vi "B_WriteClassAttribute.vi"(8 "error in (no error)":errorcluster, 11 "reference in":refnum<class "BaseTemplate_4x4x4.lvclass">) -> (0 "error out":errorcluster, 3 "reference out":refnum<class "BaseTemplate_4x4x4.lvclass">)   [LabVIEW 2012]
uses:
  <resource>/Framework/Providers/Open_GDS/ClassProviders/Provider_EndevoGOOP300/Templates/BaseTemplate_4x4x4/BaseTemplate_4x4x4.lvclass
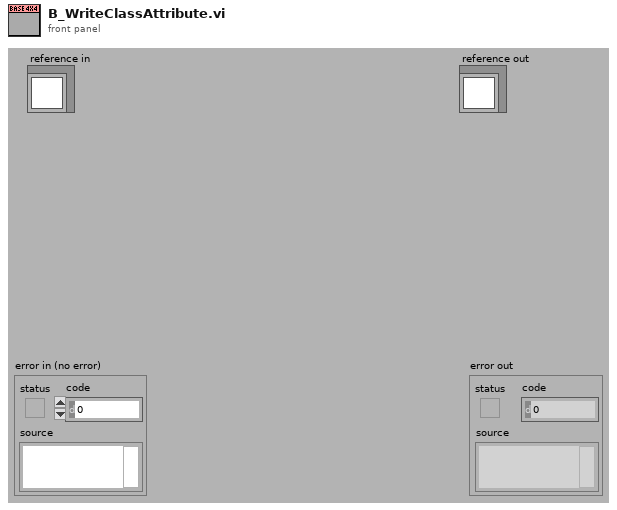
[diagram p1: front panel]
types:
  T1 = typedef "BaseTemplate_4x4x4.lvclass/ClassAttributes.ctl" = cluster{"classAttribute1":bool}
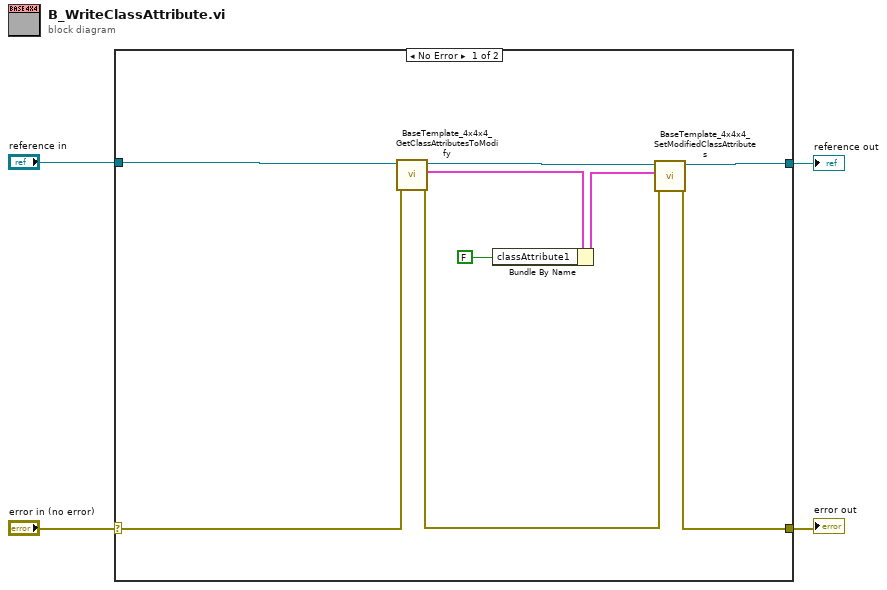
[diagram p0: block diagram]
diagram:
  n1 = case shown="No Error" "error in (no error)" {
    selector: "error in (no error)" -> [w6 w15]
    tunnel: [w10 w15] -> w3
    tunnel: [w9 w14] -> w1
    tunnel: "reference in" -> [w5 w14]
    frame No Error {
      n2 = call <resource>:"BaseTemplate_4x4x4_GetClassAttributesToModify.vi"("error in (no error)"=w6, "reference in"=w5) -> ("error out"=w8:errorcluster, "Class attributes"=w13:T1, "reference out"=w11:refnum<class "BaseTemplate_4x4x4.lvclass">)  [unwired: 6 in, 1 out]
      n3 = Bundle By Name(cluster=w13, "classAttribute1"=FALSE) -> (w12:T1)
      n4 = call <resource>:"BaseTemplate_4x4x4_SetModifiedClassAttributes.vi"("error in (no error)"=w8, "Class attributes"=w12, "reference in"=w11) -> ("error out"=w10:errorcluster, "reference out"=w9:refnum<class "BaseTemplate_4x4x4.lvclass">)  [unwired: 7 in]
    }
    frame Error {
    }
  }
  "error out" <- w3
  "reference out" <- w1
